vi "MV3D RGBD Set Ip Config.vi"(10 "pstIPConfig":T1={"enIPCfgMode"=1, "chDestIp[0]"=0, "chDestIp[1]"=0, "chDestIp[2]"=0, "chDestIp[3]"=0, "chDestIp[4]"=0, "chDestIp[5]"=0, "chDestIp[6]"=0, "chDestIp[7]"=0, "chDestIp[8]"=0, "chDestIp[9]"=0, "chDestIp[10]"=0, "chDestIp[11]"=0, "chDestIp[12]"=0, "chDestIp[13]"=0, "chDestIp[14]"=0, "chDestIp[15]"=0, "chDestNetMask[0]"=0, "chDestNetMask[1]"=0, "chDestNetMask[2]"=0, "chDestNetMask[3]"=0, "chDestNetMask[4]"=0, "chDestNetMask[5]"=0, "chDestNetMask[6]"=0, "chDestNetMask[7]"=0, "chDestNetMask[8]"=0, "chDestNetMask[9]"=0, "chDestNetMask[10]"=0, "chDestNetMask[11]"=0, "chDestNetMask[12]"=0, "chDestNetMask[13]"=0, "chDestNetMask[14]"=0, "chDestNetMask[15]"=0, "chDestGateWay[0]"=0, "chDestGateWay[1]"=0, "chDestGateWay[2]"=0, "chDestGateWay[3]"=0, "chDestGateWay[4]"=0, "chDestGateWay[5]"=0, "chDestGateWay[6]"=0, "chDestGateWay[7]"=0, "chDestGateWay[8]"=0, "chDestGateWay[9]"=0, "chDestGateWay[10]"=0, "chDestGateWay[11]"=0, "chDestGateWay[12]"=0, "chDestGateWay[13]"=0, "chDestGateWay[14]"=0, "chDestGateWay[15]"=0, "nReserved[0]"=0, "nReserved[1]"=0, "nReserved[2]"=0, "nReserved[3]"=0, "nReserved[4]"=0, "nReserved[5]"=0, "nReserved[6]"=0, "nReserved[7]"=0, "nReserved[8]"=0, "nReserved[9]"=0, "nReserved[10]"=0, "nReserved[11]"=0, "nReserved[12]"=0, "nReserved[13]"=0, "nReserved[14]"=0, "nReserved[15]"=0} {"enIPCfgMode" items=["IpCfgMode_Static"=1, "IpCfgMode_DHCP"=2, "IpCfgMode_LLA"=4]}, 11 "chSerialNumber":string) -> (2 "pstIPConfig out":T1={"enIPCfgMode"=1, "chDestIp[0]"=0, "chDestIp[1]"=0, "chDestIp[2]"=0, "chDestIp[3]"=0, "chDestIp[4]"=0, "chDestIp[5]"=0, "chDestIp[6]"=0, "chDestIp[7]"=0, "chDestIp[8]"=0, "chDestIp[9]"=0, "chDestIp[10]"=0, "chDestIp[11]"=0, "chDestIp[12]"=0, "chDestIp[13]"=0, "chDestIp[14]"=0, "chDestIp[15]"=0, "chDestNetMask[0]"=0, "chDestNetMask[1]"=0, "chDestNetMask[2]"=0, "chDestNetMask[3]"=0, "chDestNetMask[4]"=0, "chDestNetMask[5]"=0, "chDestNetMask[6]"=0, "chDestNetMask[7]"=0, "chDestNetMask[8]"=0, "chDestNetMask[9]"=0, "chDestNetMask[10]"=0, "chDestNetMask[11]"=0, "chDestNetMask[12]"=0, "chDestNetMask[13]"=0, "chDestNetMask[14]"=0, "chDestNetMask[15]"=0, "chDestGateWay[0]"=0, "chDestGateWay[1]"=0, "chDestGateWay[2]"=0, "chDestGateWay[3]"=0, "chDestGateWay[4]"=0, "chDestGateWay[5]"=0, "chDestGateWay[6]"=0, "chDestGateWay[7]"=0, "chDestGateWay[8]"=0, "chDestGateWay[9]"=0, "chDestGateWay[10]"=0, "chDestGateWay[11]"=0, "chDestGateWay[12]"=0, "chDestGateWay[13]"=0, "chDestGateWay[14]"=0, "chDestGateWay[15]"=0, "nReserved[0]"=0, "nReserved[1]"=0, "nReserved[2]"=0, "nReserved[3]"=0, "nReserved[4]"=0, "nReserved[5]"=0, "nReserved[6]"=0, "nReserved[7]"=0, "nReserved[8]"=0, "nReserved[9]"=0, "nReserved[10]"=0, "nReserved[11]"=0, "nReserved[12]"=0, "nReserved[13]"=0, "nReserved[14]"=0, "nReserved[15]"=0} {"enIPCfgMode" items=["IpCfgMode_Static"=1, "IpCfgMode_DHCP"=2, "IpCfgMode_LLA"=4]}, 3 "function return":i32)   [LabVIEW 2015, in "Mv3dRgbd.lvlib"]
doc: "MV3D_RGBD_API MV3D_RGBD_STATUS MV3D_RGBD_SetIpConfig(const char* chSerialNumber, MV3D_RGBD_IP_CONFIG* pstIPConfig);"
uses:
  <userlib>/Mv3dRgbd/Mv3dRgbd.lvlib
  <userlib>/Mv3dRgbd/Mv3dRgbd.dll
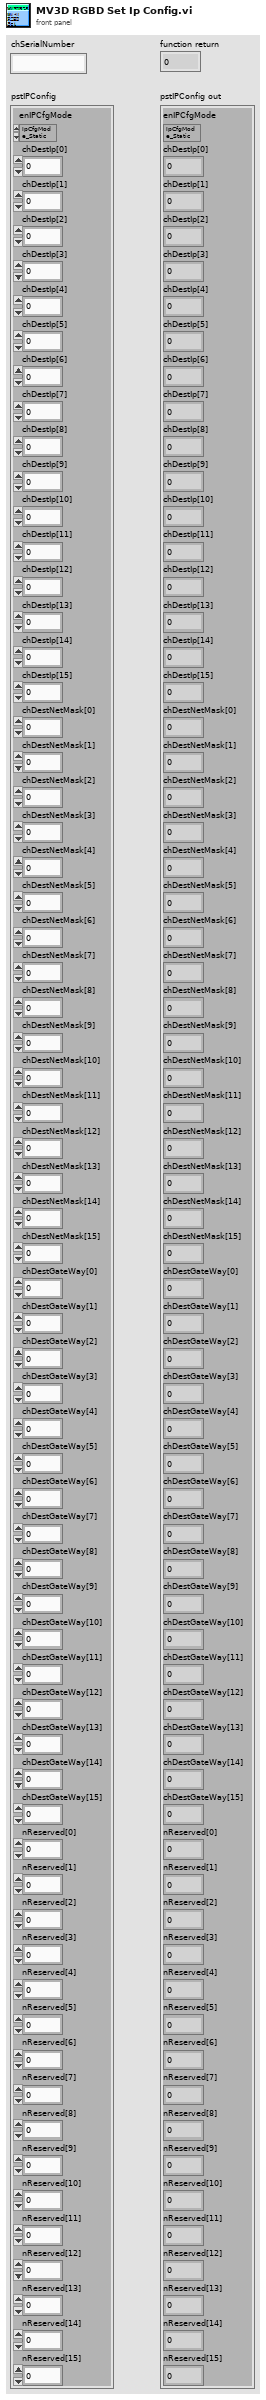
[diagram p1: front panel]
types:
  T1 = cluster{"enIPCfgMode":u32, "chDestIp[0]":i8, "chDestIp[1]":i8, "chDestIp[2]":i8, "chDestIp[3]":i8, "chDestIp[4]":i8, "chDestIp[5]":i8, "chDestIp[6]":i8, "chDestIp[7]":i8, "chDestIp[8]":i8, "chDestIp[9]":i8, "chDestIp[10]":i8, "chDestIp[11]":i8, "chDestIp[12]":i8, "chDestIp[13]":i8, "chDestIp[14]":i8, "chDestIp[15]":i8, "chDestNetMask[0]":i8, "chDestNetMask[1]":i8, "chDestNetMask[2]":i8, "chDestNetMask[3]":i8, "chDestNetMask[4]":i8, "chDestNetMask[5]":i8, "chDestNetMask[6]":i8, "chDestNetMask[7]":i8, "chDestNetMask[8]":i8, "chDestNetMask[9]":i8, "chDestNetMask[10]":i8, "chDestNetMask[11]":i8, "chDestNetMask[12]":i8, "chDestNetMask[13]":i8, "chDestNetMask[14]":i8, "chDestNetMask[15]":i8, "chDestGateWay[0]":i8, "chDestGateWay[1]":i8, "chDestGateWay[2]":i8, "chDestGateWay[3]":i8, "chDestGateWay[4]":i8, "chDestGateWay[5]":i8, "chDestGateWay[6]":i8, "chDestGateWay[7]":i8, "chDestGateWay[8]":i8, "chDestGateWay[9]":i8, "chDestGateWay[10]":i8, "chDestGateWay[11]":i8, "chDestGateWay[12]":i8, "chDestGateWay[13]":i8, "chDestGateWay[14]":i8, "chDestGateWay[15]":i8, "nReserved[0]":u8, "nReserved[1]":u8, "nReserved[2]":u8, "nReserved[3]":u8, "nReserved[4]":u8, "nReserved[5]":u8, "nReserved[6]":u8, "nReserved[7]":u8, "nReserved[8]":u8, "nReserved[9]":u8, "nReserved[10]":u8, "nReserved[11]":u8, "nReserved[12]":u8, "nReserved[13]":u8, "nReserved[14]":u8, "nReserved[15]":u8}
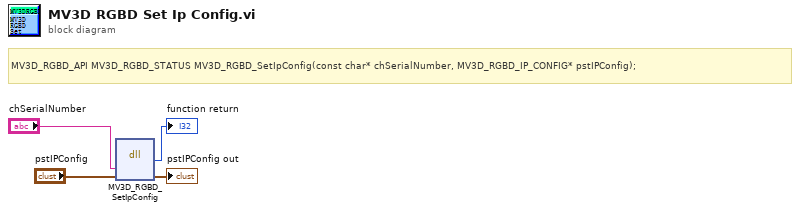
[diagram p0: block diagram]
diagram:
  # "MV3D_RGBD_API MV3D_RGBD_STATUS MV3D_RGBD_SetIpConfig(const char* chSerialNumber, MV3D_RGBD_IP_CONFIG* pstIPConfig);"
  n1 = dll-call lib="C:/Program Files (x86)/National Instruments/LabVIEW 2015/user.lib/Mv3dRgbd/Mv3dRgbd.*" fn="MV3D_RGBD_SetIpConfig"("chSerialNumber"="chSerialNumber", "pstIPConfig"="pstIPConfig") -> (→"function return":i32, "pstIPConfig"=→"pstIPConfig out":T1)  [unwired: 4 in, 2 out]
